vi "Test3v5.vi"() -> ()   [LabVIEW 2013]
panel:
  out "unsigned byte array":u8[](array[numeric])
  out "*(type *) &x 2":string
  out "String":string
  out "subarray":string[](array[string])
  out "index":i32
  out "*(type *) &x":string
  out "size(s)":i32
  out "hex integer string":string[](array[string])
  in  "error in":errorcluster
  out "error out":errorcluster
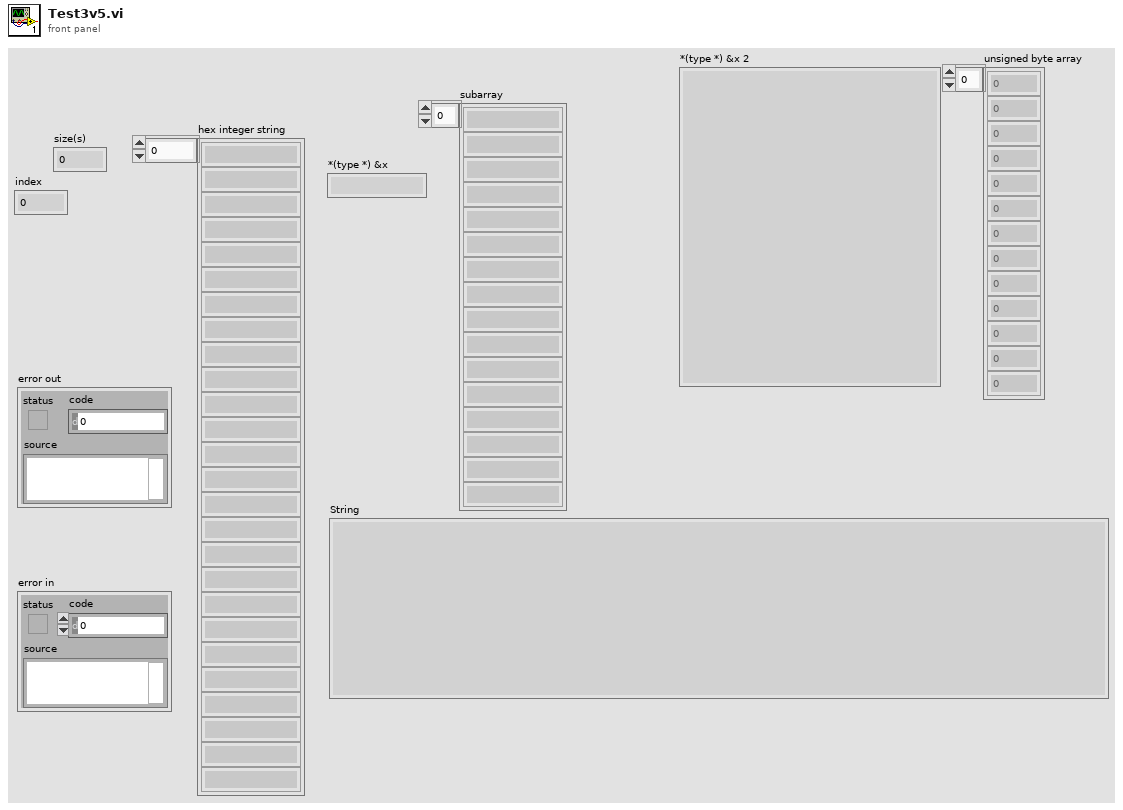
[diagram p1: front panel]
types:
  T1 = enum16{"big-endian, network order", "native, host order", "little-endian"}
  T2 = enum16{"open", "replace", "create", "open or create", "replace or create", "replace or create with confirmation"}
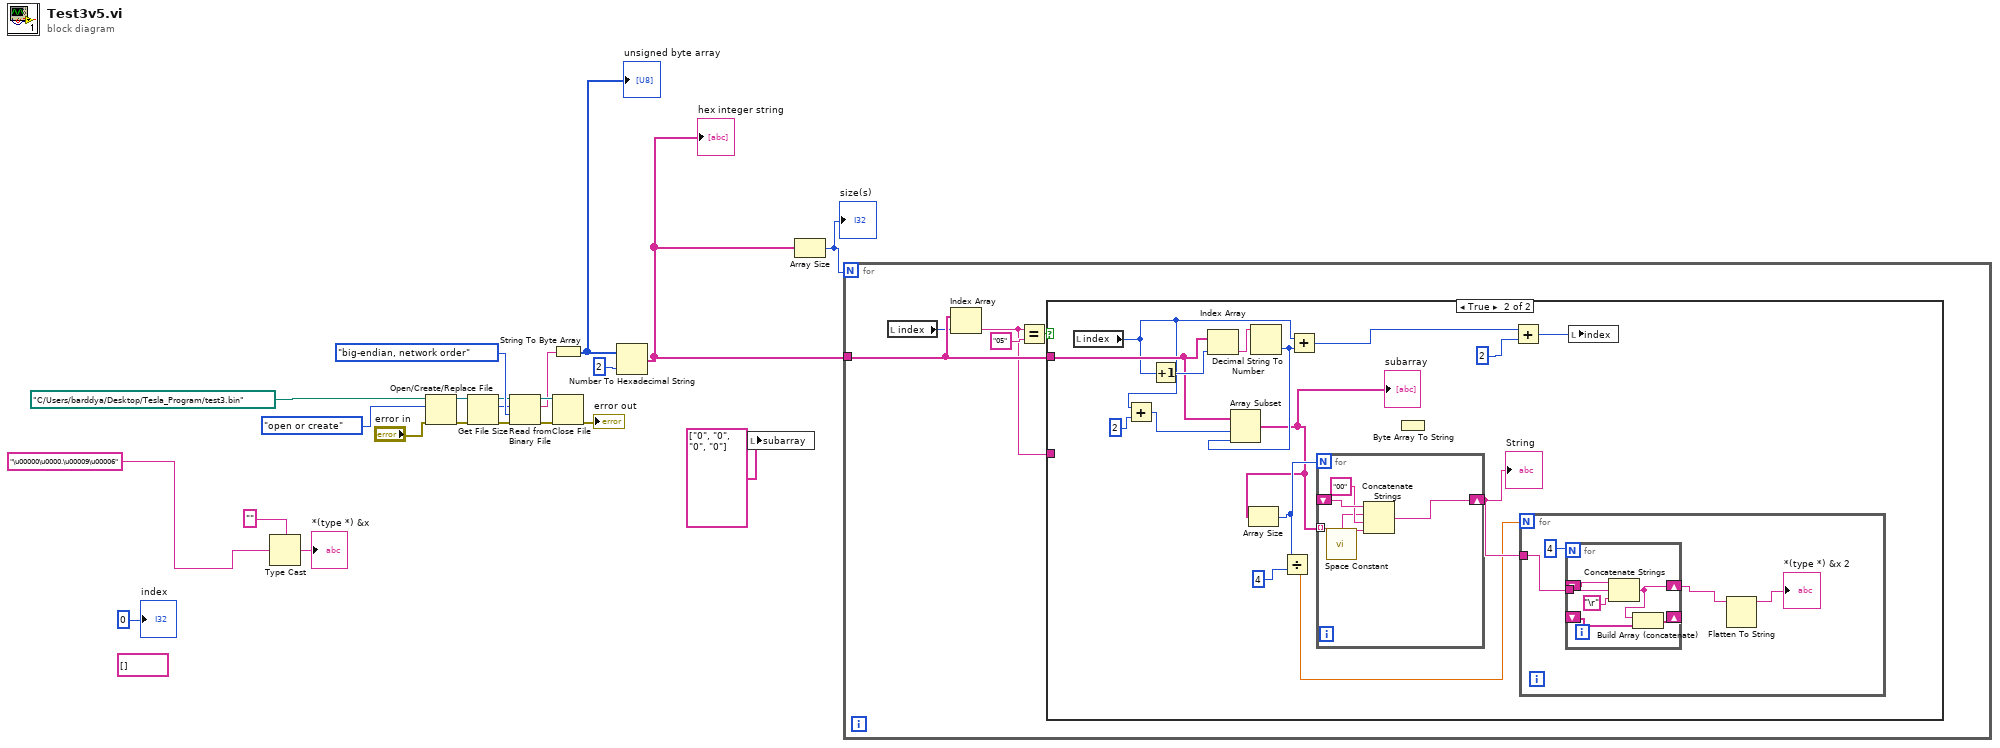
[diagram p0: block diagram]
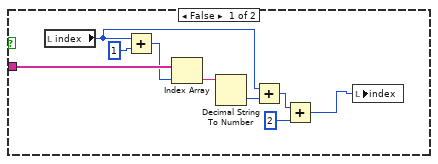
[diagram p2: hidden frame]
diagram:
  (unwired) string[] [] ("subarray")
  n1 = Type Cast(type="", x="\u00000\u0000.\u00009\u00006") -> (*(type *) &x=→"*(type *) &x":string)
  n2 = Open/Create/Replace File(file path (use dialog)=path "C:/Users/barddya/Desktop/Tesla_Program/test3.bin", error in="error in", operation (0:open)=T2."open or create") -> (refnum out=w15:refnum<file>, error out=w13:errorcluster)  [unwired: 3 in, 1 out]
  n3 = Get File Size(file=w15, error in=w13) -> (refnum out=w14:refnum<file>, size (in bytes)=w11:i64, 0:w12:errorcluster)
  n4 = Read from Binary File(8:w12, 9:T1."big-endian, network order" ("byte order (0:big-endian, network order)"), 10:w11, 11:w14) -> (0:w18:errorcluster, 2:w10:string, 3:w16:refnum<file>)  [unwired: 2 in, 1 out]
  n5 = String To Byte Array(string=w10) -> (unsigned byte array=w9:u8[])
  "unsigned byte array" <- w9
  n6 = Close File(refnum=w16, error in=w18) -> (error out=→"error out":errorcluster)  [unwired: 1 out]
  n7 = Number To Hexadecimal String(1:2, 2:w9) -> (0:w1:string[])
  "hex integer string" <- w1
  n8 = local write "subarray"(string[] ["0", "0", "0", "0"] ("subarray")) -> ()
  n9 = Array Size(array=w1) -> (size(s)=w4:i32)
  "size(s)" <- w4
  n10 = for {
    N: w4 -> [_]
    tunnel: w1 -> [w25]
    n11 = local read "index"() -> (w23:i32)
    n12 = Index Array(array=w25, index=w23) -> (element=w24:string)
    n13 = Equal?(x=w24, y="05") -> (x = y?=w26:bool)
    n14 = case shown="True" w26 {
      tunnel: w25 -> [w34 w48]
      tunnel: w24 -> [_ _]
      frame False {
        n15 = local read "index"() -> (w31:i32)
        n16 = Add(x=w31, y=1) -> (x+y=w32:i32)
        n17 = Index Array(array=w34, index=w32) -> (element=w36:string)
        n18 = Decimal String To Number(string=w36) -> (number=w35:i32)  [unwired: 2 in, 1 out]
        n19 = Add(x=w31, y=w35) -> (x+y=w30:i32)
        n20 = Add(x=w30, y=2) -> (x+y=w28:i32)
        n21 = local write "index"(w28) -> ()
      }
      frame True {
        n22 = local read "index"() -> (w46:i32)
        n23 = Add(x=w46, y=2) -> (x+y=w44:i32)
        n24 = Increment(x=w46) -> (x+1=w51:i32)
        n25 = Index Array(array=w48, index=w51) -> (element=w49:string)
        n26 = Decimal String To Number(string=w49) -> (number=w42:i32)  [unwired: 2 in, 1 out]
        n27 = Array Subset(array=w48, index=w44, length=w42) -> (w37:string[])
        "subarray" <- w37
        n28 = Array Size(array=w37) -> (size(s)=w40:i32)
        n29 = Divide(x=w40, y=4) -> (x/y=w38:dbl)
        n30 = Add(x=w46, y=w42) -> (x+y=w47:i32)
        n31 = for {
          N: w40 -> [_]
          tunnel: w37 -> [w65] mode=indexing
          shift-right: [w66] -> w41
          shift-left: _ -> [w64]
          n32 = call <vilib>:"Space Constant.vi"() -> ("String"=w62:string)
          n33 = Concatenate Strings(w64, w62, "00", w65) -> (w66:string)
        }
        "String" <- w41
        n34 = Byte Array To String() -> ()  [unwired: 1 in, 1 out]
        n35 = Add(x=w47, y=2) -> (x+y=w43:i32)
        n36 = for {
          N: w38 -> [_]
          tunnel: w41 -> [w54]
          n37 = for {
            N: 4 -> [_]
            shift-right: [w61] -> _
            shift-left: _ -> [w60]
            shift-right: [w59] -> w53
            shift-left: _ -> [w58]
            tunnel: w54 -> [w57]
            n38 = Concatenate Strings(w58, w57, "\r") -> (w59:string)
            n39 = Build Array (concatenate)(w59, w60) -> (w61:string[])
          }
          n40 = Flatten To String(anything=w53) -> (data string=→"*(type *) &x 2":string)  [unwired: 3 in, 2 out]
        }
        n41 = local write "index"(w43) -> ()
      }
    }
  }
  "index" <- 0
